vi "Save Data.vi"(4 "PI<0> Measurements":T2={"voltage measurements"=[200.0], "current measurements"=[201.0]} {"current measurements" format="%#_6p"}, 6 "HV Measurements":T2={"voltage measurements"=[100.0], "current measurements"=[101.0]} {"current measurements" format="%#_6p"}, 8 "Error In":errorcluster, 9 "Dut and Bridge Measurements":T2={"voltage measurements"=[90.0, 91.0, 92.0, 93.0], "current measurements"=[80.0, 81.0, 82.0, 83.0]} {"current measurements" format="%#_6p"}, 10 "DUT Info":T1={"Lot #"="12345", "Wafer #"="54321", "DUT Coordinates"="22_13", "Comments"="experimant"}, 11 "Path":path) -> (0 "error out":errorcluster)   [LabVIEW 2013]
uses:
  <vilib>/Utility/file.llb/Write To Spreadsheet File (string).vi
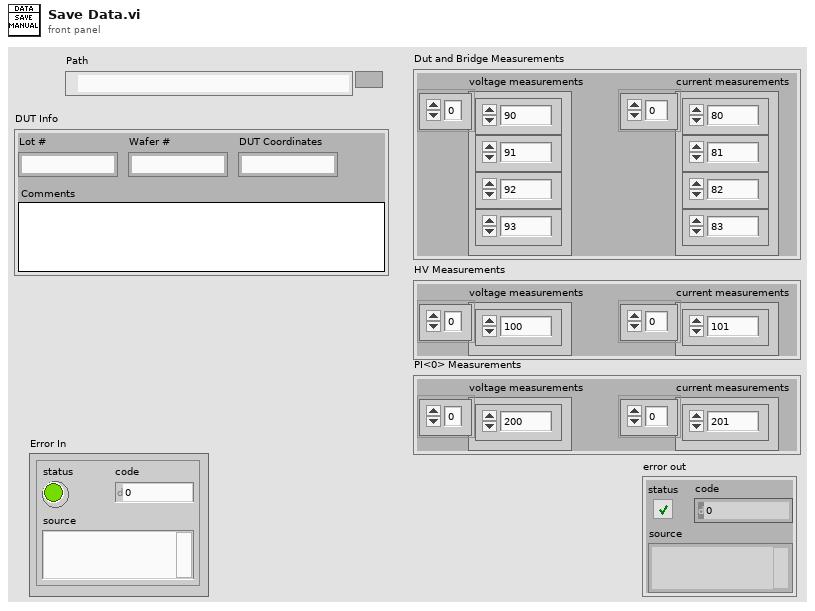
[diagram p1: front panel]
types:
  T1 = cluster{"Lot #":string, "Wafer #":string, "DUT Coordinates":string, "Comments":string}
  T2 = cluster{"voltage measurements":dbl[], "current measurements":dbl[]}
  T3 = cluster{"voltage measurements":dbl[], "current measurements":dbl[]}[]
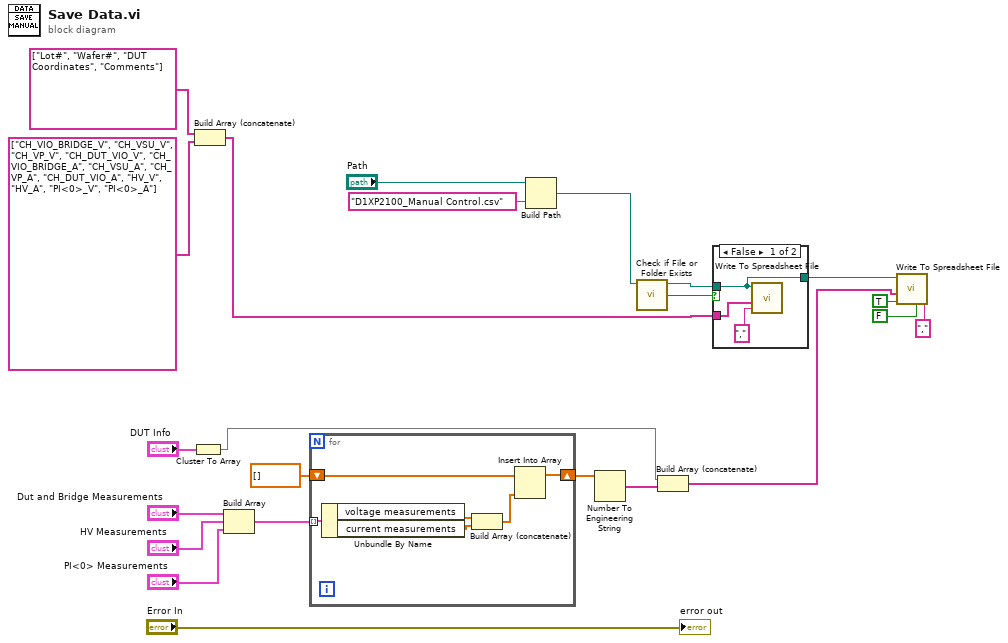
[diagram p0: block diagram]
diagram:
  n1 = Cluster To Array(cluster="DUT Info") -> (array=w3:string[])
  n2 = Build Array (concatenate)(string[] ["Lot#", "Wafer#", "DUT Coordinates", "Comments"], string[] ["CH_VIO_BRIDGE_V", "CH_VSU_V", "CH_VP_V", "CH_DUT_VIO_V", "CH_VIO_BRIDGE_A", "CH_VSU_A", "CH_VP_A", "CH_DUT_VIO_A", "HV_V", "HV_A", "PI<0>_V", "PI<0>_A"]) -> (w11:string[])
  n3 = Build Array("Dut and Bridge Measurements", "HV Measurements", "PI<0> Measurements") -> (w20:T3)
  n4 = for {
    tunnel: w20 -> [w29] mode=indexing
    shift-right: [w25] -> w5
    shift-left: dbl[] [] -> [w24]
    n5 = Unbundle By Name(w29) -> ("voltage measurements"=w28:dbl[], "current measurements"=w27:dbl[])
    n6 = Build Array (concatenate)(w28, w27) -> (w26:dbl[])
    n7 = Insert Into Array(array=w24, new element=w26) -> (w25:dbl[])  [unwired: 1 in]
  }
  n8 = Build Path(base path="Path", name or relative path="D1XP2100_Manual Control.csv") -> (appended path=w8:path)
  n9 = Number To Engineering String(4:w5) -> (0:w4:string[])  [unwired: 3 in]
  n10 = call <vilib>:"Check if File or Folder Exists.vi"("path"=w8) -> ("file or folder exists?"=w16:bool, "dup path"=w15:path)  [unwired: 8 in, 1 out]
  n11 = Build Array (concatenate)(w3, w4) -> (w2:string[])
  n12 = case shown="False" w16 {
    tunnel: w15 -> [w30 w33]
    tunnel: w11 -> [w32 _]
    tunnel: [w30 w33] -> w10
    frame False {
      n13 = call-poly <vilib>:"Write To Spreadsheet File.vi"("delimiter (\\t)"="," ("delimiter (\\t)"), "1D data"=w32, "file path (dialog if empty)"=w30) -> ()  [unwired: 5 in, 1 out]
    }
    frame True {
    }
  }
  n14 = call-poly <vilib>:"Write To Spreadsheet File.vi"("delimiter (\\t)"="," ("delimiter (\\t)"), "transpose? (no:F)"=FALSE, "append to file? (new file:F)"=TRUE, "1D data"=w2, "file path (dialog if empty)"=w10) -> ()  [unwired: 3 in, 1 out]
  "error out" <- "Error In"
